vi "Get Triggered Log State.vi"(8 "error in (no error)":errorcluster, 11 "Triggered Log in":refnum<class "Triggered Log.lvclass">) -> (0 "error out":errorcluster, 2 "Triggered Log State":T1, 3 "Triggered Log out":refnum<class "Triggered Log.lvclass">)   [LabVIEW 2015, in "Triggered Log.lvclass"]
uses:
  Triggered Log.lvclass
  Triggered Log State.ctl
  Triggered Log.lvclass/Triggered Log.ctl
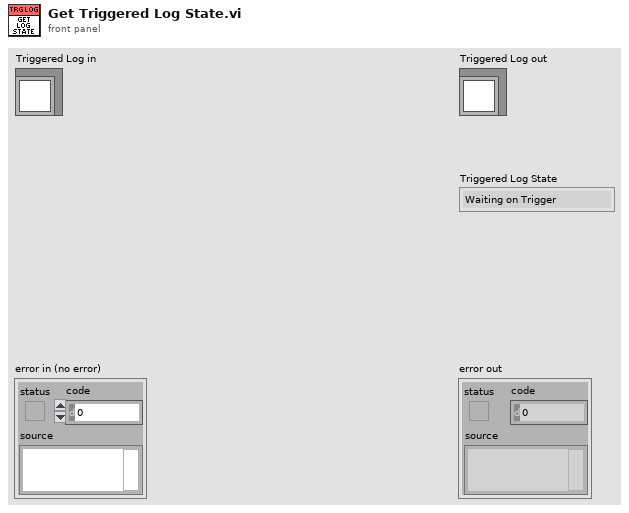
[diagram p1: front panel]
types:
  T1 = typedef "Triggered Log.lvclass/Triggered Log State.ctl" = enum16{"Waiting on Trigger", "Triggered", "Posttrigger", "Complete", "Idle", "Error"}
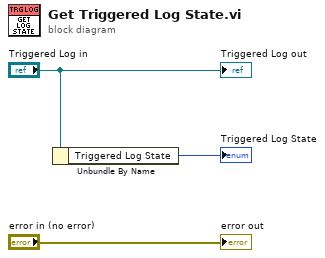
[diagram p0: block diagram]
diagram:
  n1 = Unbundle By Name("Triggered Log in") -> ("Triggered Log State"=→"Triggered Log State":T1)
  "error out" <- "error in (no error)"
  "Triggered Log out" <- "Triggered Log in"
